vi "ASK-MOD.vi"() -> ()   [LabVIEW 2012]
uses:
  <vilib>/express/express analysis/Spectral/Block/exnSpectralBlock spectral measurements peak poly.vi
  <vilib>/express/express analysis/Spectral/Block/exnSpectralBlock spectral measurements peak DDT.vi
  <vilib>/express/express analysis/Spectral/XNode/ExpressSpectralMeasurementsBlockNode.xnode
panel:
  in  "fc":dbl(slide) scale=0.0..1000.0
  in  "fm":dbl(slide) scale=0.0..500.0
  out "Waveform Graph 2":dynamicdata(graph)
  out "Modulated Graph":dynamicdata(graph)
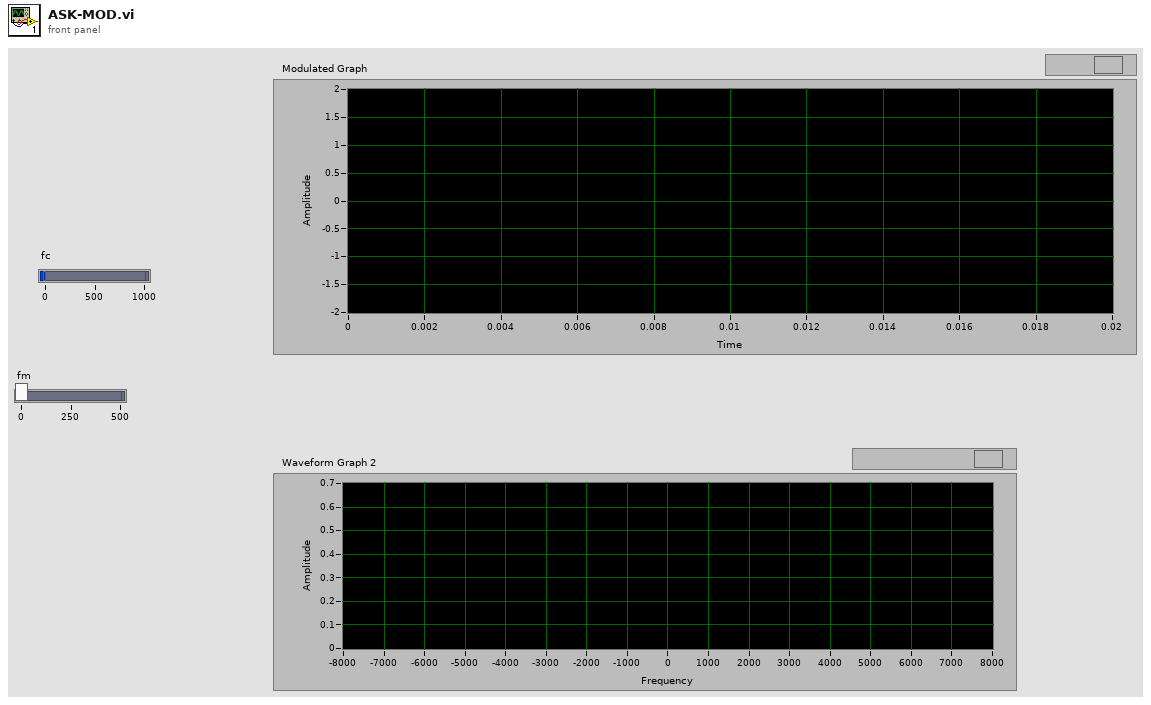
[diagram p1: front panel]
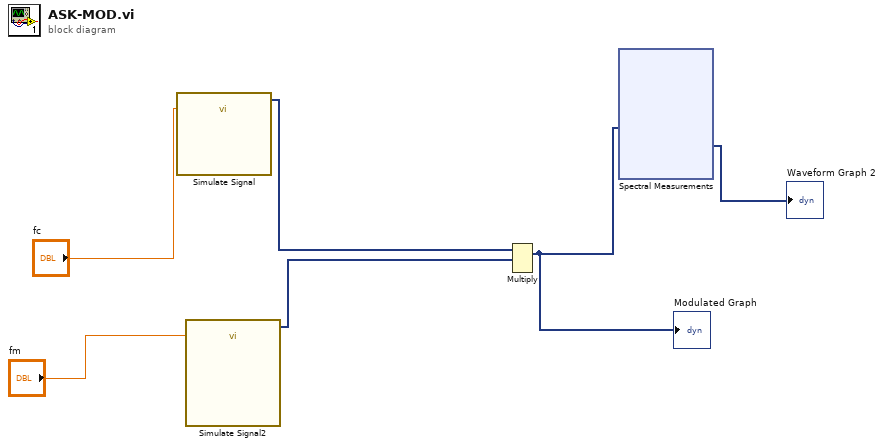
[diagram p0: block diagram]
diagram:
  n1 = call "Simulate Signal"("Frequency"="fc") -> ("Sine"=w6:dynamicdata)  [unwired: 13 in, 1 out]
  n2 = call "Simulate Signal2"("Frequency"="fm") -> ("Square"=w5:dynamicdata)  [unwired: 13 in, 1 out]
  n3 = Multiply(1:w5, 2:w6) -> (0:w4:dynamicdata)  [unwired: 1 in, 1 out]
  "Modulated Graph" <- w4
  n4 = xnode "Spectral Measurements"("Signals"=w4) -> ("FFT - (Peak)"=→"Waveform Graph 2":dynamicdata)  [unwired: 1 in, 2 out]
